vi "Main UI.vi"() -> ()   [LabVIEW 2009, in "UI.lvlib"]
uses:
  UI.lvlib
  Close Notification.vi
  Experiments UI.vi
panel:
  in  "Tab Control":enum32{"Experiment Control", "Page 2"}(tab)
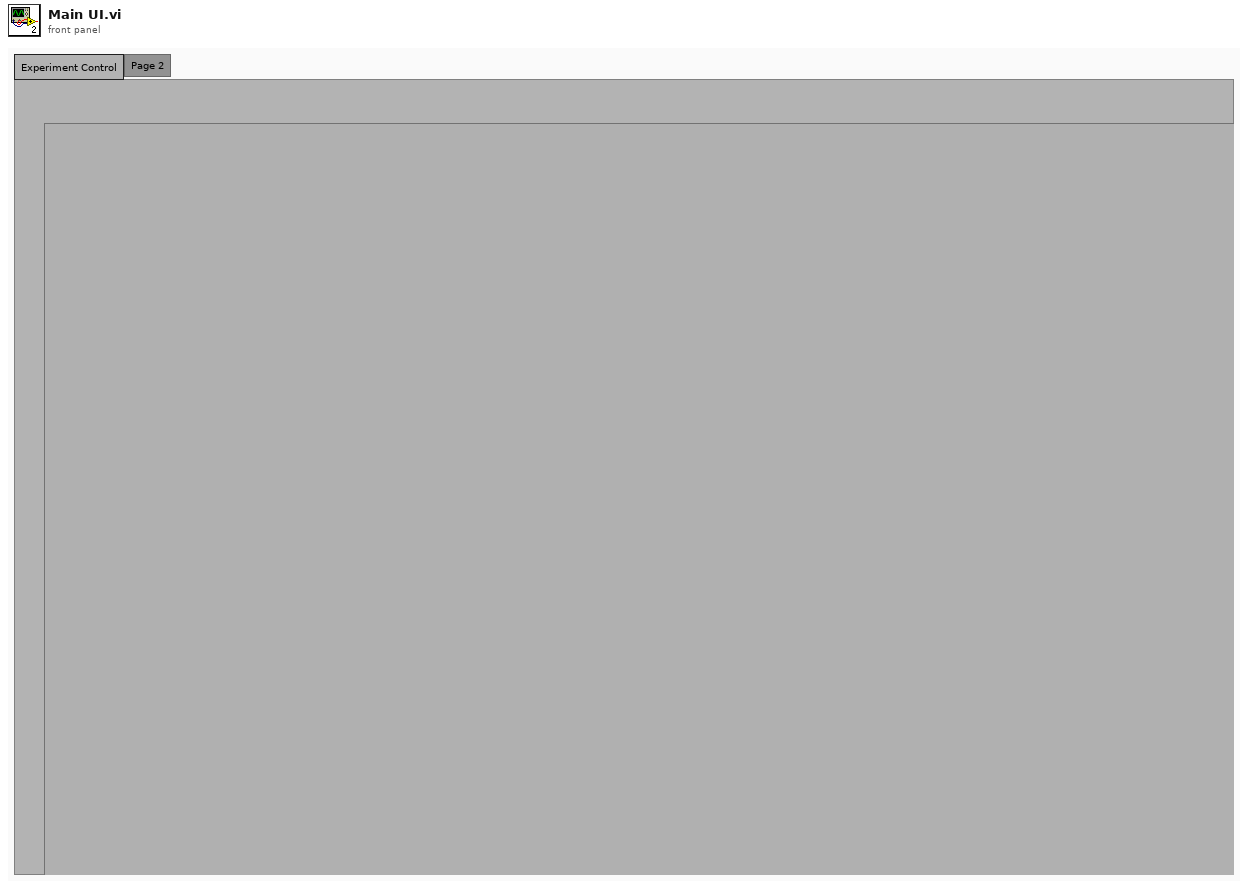
[diagram p1: front panel]
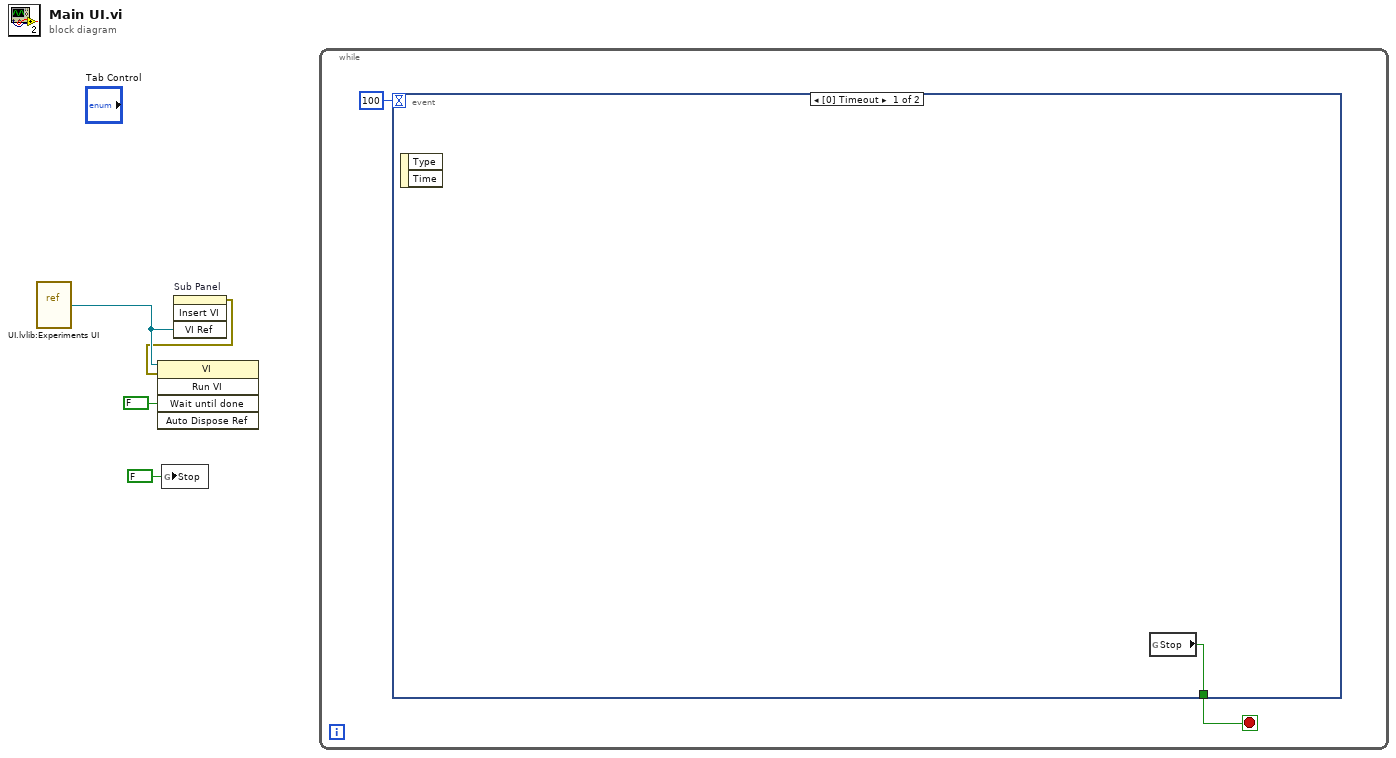
[diagram p0: block diagram]
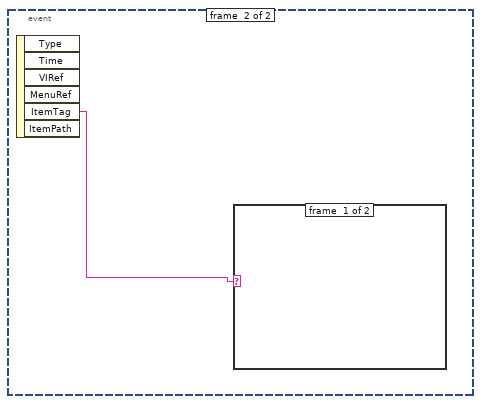
[diagram p2: hidden frame]
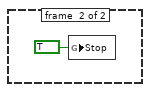
[diagram p3: hidden frame]
diagram:
  n1 = vi-ref "UI.lvlib:Experiments UI.vi"() -> (w4:refnum<vi>)
  n2 = global write "Close Notification.vi" "Stop"(FALSE ("Stop")) -> ()
  n3 = invoke on="Sub Panel" class="SubPnl" method="Insert VI"("VI Ref"=w4) -> (error out=w3:errorcluster)  [unwired: 3 in, 3 out]
  n4 = invoke class="VI" method="Run VI"(reference=w4, error in=w3, "Wait until done"=FALSE ("Wait Until Done")) -> ()  [unwired: 2 in, 5 out]
  n5 = while {
    stop <- w5 stop-if-true
    n6 = event shown="[0] Timeout" {
      selector: _ -> [_ _]
      dyn-events: _ -> [_ _]
      timeout: 100 -> [_ _]
      tunnel: [w7 _] -> w5
      event #0 {
        n7 = event-data() -> ()  [unwired: 1 in, 2 out]
        n8 = global read "Close Notification.vi" "Stop"() -> (w7:bool)
      }
      event #1 {
        n9 = event-data() -> ("ItemTag"=w8:string)  [unwired: 1 in, 5 out]
        n10 = case shown="\"False\", Default" w8 {
          frame #0 {
          }
          frame #1 {
            n11 = global write "Close Notification.vi" "Stop"(TRUE ("Stop")) -> ()
          }
        }
      }
    }
  }
